vi "resistanceCheck.vi"() -> ()   [LabVIEW 2018]
panel:
  out "Array 2":dbl[](array[numeric])
  out "continuousADC":dbl
  in  "stop 2":bool
  out "stepICON":dbl
  out "buttonADC":dbl
  out "Ipeak":string
  out "result":bool
  in  "stop":bool
  out "overCurrent":bool
  out "resistance":cluster{dbl, dbl}(graph)
  out "upper":u32
  out "lower":u32
  out "button":dbl
  out "Array":dbl[](array[numeric])
  out "cycle":dbl
  out "ICON":cluster{dbl, dbl}[](array[cluster])
  out "steps/button Array":dbl[][](array[numeric])
  out "KeyCodeName":string[](array[string])
  in  "VISA resource name":refnum<visa-resource-name>
  out "EQF1255":cluster{dbl, dbl}[](array[cluster])
  out "step":dbl
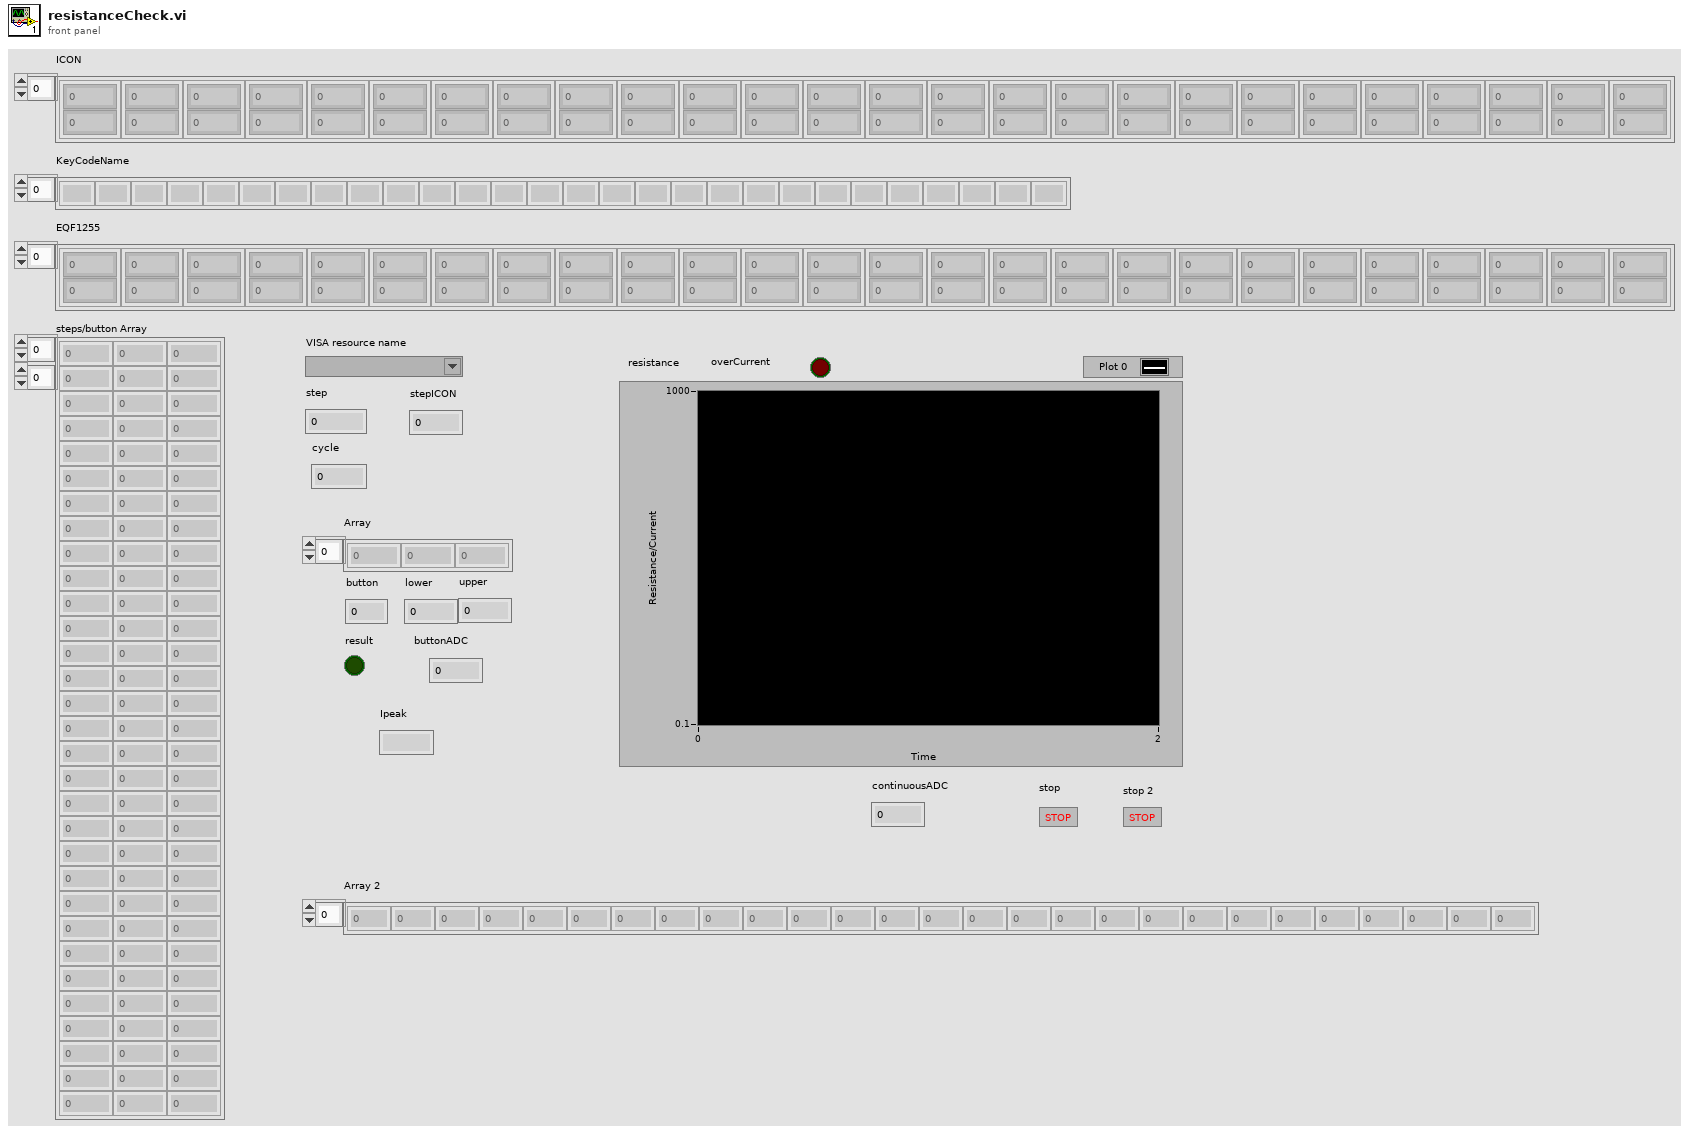
[diagram p1: front panel]
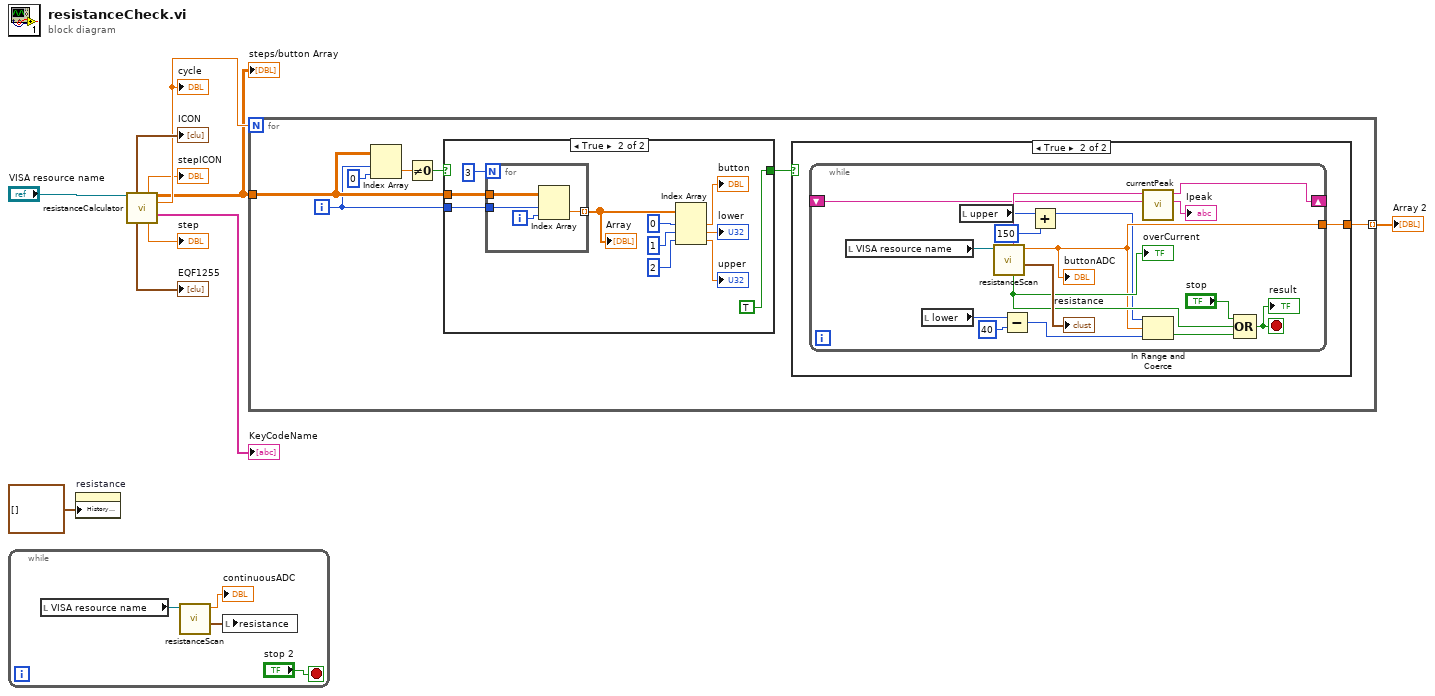
[diagram p0: block diagram]
diagram:
  n1 = while {
    stop <- "stop 2" stop-if-true
    n2 = local read "VISA resource name"() -> (w14:refnum<visa-resource-name>)
    n3 = call "resistanceScan.vi"("VISA Refnum in"=w14) -> ("RESISTANCE/CURRENT"=w11:cluster{dbl, dbl}, "ADC value"=→"continuousADC":dbl)  [unwired: 6 in, 3 out]
    n4 = local write "resistance"(w11) -> ()
  }
  n5 = property on="resistance" class="WFChart (strict)"("History Data"=cluster{dbl, dbl}[] []) -> ()  [unwired: 2 in, 2 out]
  n6 = call "resistanceCalculator.vi"("VISA Refnum in"="VISA resource name") -> ("ICON"=→"ICON":cluster{dbl, dbl}[], "stepICON"=→"stepICON":dbl, "steps/button Array"=w6:dbl[][], "cycle"=w7:dbl, "KeyCodeName"=→"KeyCodeName":string[], "EQF1255"=→"EQF1255":cluster{dbl, dbl}[], "stepEQF1255"=→"step":dbl)  [unwired: 6 in, 2 out]
  "steps/button Array" <- w6
  "cycle" <- w7
  n7 = for {
    N: w7 -> [_]
    tunnel: w6 -> [w20]
    tunnel: [w15] -> w3 mode=indexing
    i -> [w19]
    n8 = Index Array(array=w20, index (row)=w19, index (col)=0 ("disabled index (col)")) -> (element=w21:dbl)
    n9 = Not Equal To 0?(x=w21) -> (x != 0?=w17:bool)
    n10 = case shown="True" w17 {
      selector: w17 -> [w40 _]
      tunnel: w20 -> [_ w50]
      tunnel: w19 -> [_ w49]
      tunnel: [w40 TRUE] -> w16
      frame False {
      }
      frame True {
        n11 = for {
          N: 3 -> [_]
          tunnel: w50 -> [w55]
          tunnel: [w54] -> w48 mode=indexing
          tunnel: w49 -> [w53]
          i -> [w52]
          n12 = Index Array(array=w55, index (row)=w53, index (col)=w52) -> (element=w54:dbl)
        }
        "Array" <- w48
        n13 = Index Array(array=w48, index #1=0 ("index"), index #2=1 ("index"), index #3=2 ("index")) -> (element #1=→"button":dbl, element #2=→"lower":dbl, element #3=→"upper":dbl)
      }
    }
    n14 = case shown="True" w16 {
      tunnel: [_ w22] -> w15
      frame False {
      }
      frame True {
        n15 = while {
          shift-right: [w31] -> _
          shift-left: _ -> [w30]
          tunnel: [w26] -> w22
          stop <- w35 stop-if-true
          n16 = local read "VISA resource name"() -> (w39:refnum<visa-resource-name>)
          n17 = local read "lower"() -> (w37:u32)
          n18 = local read "upper"() -> (w24:u32)
          n19 = call "resistanceScan.vi"("VISA Refnum in"=w39) -> ("RESISTANCE/CURRENT"=→"resistance":cluster{dbl, dbl}, "ADC value"=w26:dbl, "overCurrent"=w34:bool, "Istring#"=w32:string)  [unwired: 6 in, 1 out]
          "overCurrent" <- w34
          "buttonADC" <- w26
          n20 = Subtract(x=w37, y=u32 40) -> (x-y=w28:u32)
          n21 = Add(x=w24, y=u32 150) -> (x+y=w25:u32)
          n22 = call "currentPeak.vi"("Istring# change"=w30, "Istring# scan"=w32) -> ("Ipeak"=→"Ipeak":string, "Irun"=w31:string)  [unwired: 7 in, 1 out]
          n23 = In Range and Coerce(upper limit=w25, x=w26, lower limit=w28) -> (In Range?=w36:bool)  [unwired: 1 out]
          n24 = Compound Arithmetic op=OR("stop", w34, w36) -> (w35:bool)
          "result" <- w35
        }
      }
    }
  }
  "Array 2" <- w3
